vi "nipkg-updateControlFileMetadata.vi"() -> ()   [LabVIEW 2014, in "nipkg-build-system.lvlib"]
uses:
  nipkg-build-system.lvlib
  types/Package data.ctl
  <vilib>/Utility/file.llb/Read From Spreadsheet File (string).vi
  <vilib>/Utility/file.llb/Write To Spreadsheet File (string).vi
  <vilib>/Wiresmith Technology/LabVIEW CLI/CLI Class/CLI.lvclass
panel:
  out "error out":errorcluster
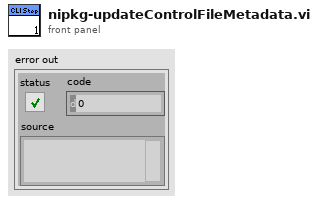
[diagram p1: front panel]
types:
  T1 = typedef "nipkg-build-system.lvlib/Package data.ctl" = cluster{"Package control file path":path, "Package metadata":string[]}
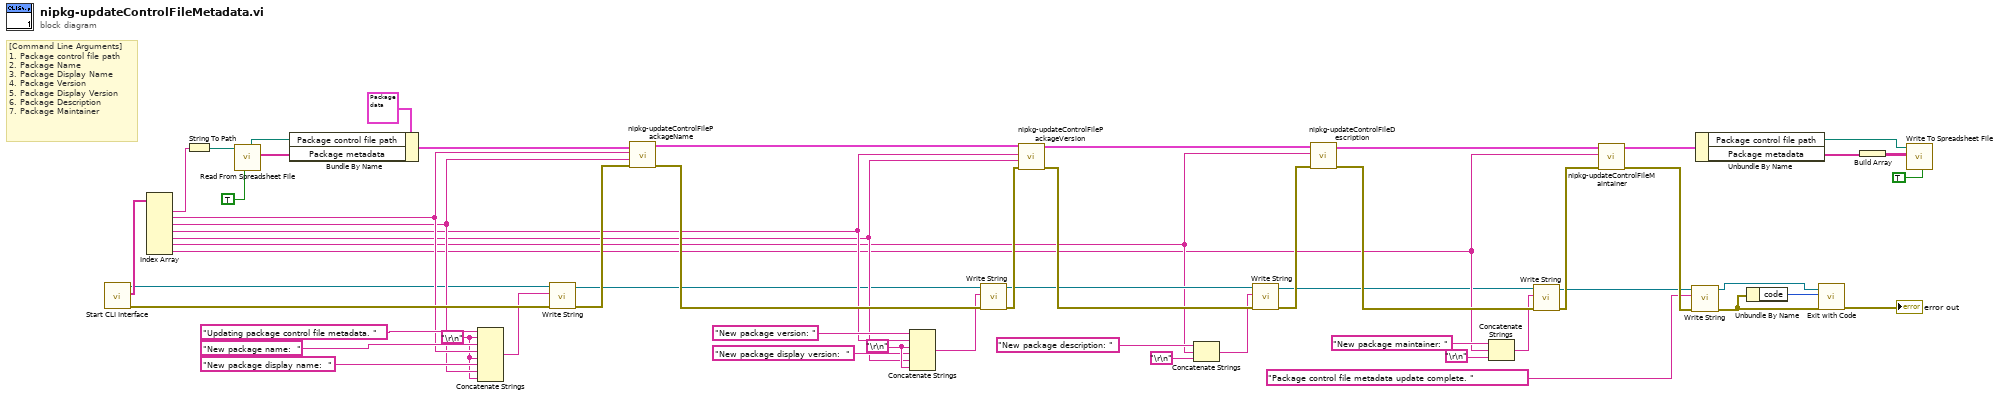
[diagram p0: block diagram]
diagram:
  w30 = "\r\n"
  w28 = "\r\n"
  # "[Command Line Arguments]\n1. Package control file path\n2. Package Name\n3. Package Display Name\n4. Package Version\n5. Package Display Version\n6. Package Description\n7. Package Maintainer"
  n1 = call <vilib>:"Start CLI Interface.vi"() -> ("error out"=w40:errorcluster, "Custom Parameters"=w43:string[], "CLI out"=w32:refnum<class "CLI.lvclass">)  [unwired: 9 in]
  n2 = Index Array(array=w43) -> (element #1=w42:string, element #2=w36:string, element #3=w34:string, element #4=w26:string, element #5=w25:string, element #6=w17:string, element #7=w12:string)  [unwired: 7 in]
  n3 = String To Path(string=w42) -> (path=w41:path)
  n4 = call-poly <vilib>:"Read From Spreadsheet File.vi"("transpose (no:F)"=TRUE, "file path (dialog if empty)"=w41) -> ("first row"=w54:string[], "new file path (Not A Path if cancelled)"=w48:path)  [unwired: 5 in, 3 out]
  n5 = Bundle By Name(cluster=T1 {"Package control file path"=path "C:/J/workspace/Waveform-Processing-CD/Package/Source/waveform-processing-custom-device/control/control", "Package metadata"=["Package: waveform-processing-custom-device"]} ("Package data"), "Package control file path"=w48, "Package metadata"=w54) -> (w53:T1)
  n6 = Concatenate Strings("Updating package control file metadata. ", w28, "New package name:  ", w36, w28, "New package display name:  ", w34, w28) -> (w33:string)
  n7 = call <vilib>:"Write String.vi"("error in (no error)"=w40, "Text to Write"=w33, "CLI in"=w32) -> ("error out"=w39:errorcluster, "CLI out"=w23:refnum<class "CLI.lvclass">)  [unwired: 7 in]
  n8 = call "nipkg-updateControlFilePackageName.vi"("error in (no error)"=w39, "New Package Display Name"=w34, "New Package Name"=w36, "Package data"=w53) -> ("error out"=w31:errorcluster, "Package data out"=w52:T1)  [unwired: 6 in]
  n9 = Concatenate Strings("New package version: ", w26, w30, "New package display version:  ", w25, w30) -> (w24:string)
  n10 = call <vilib>:"Write String.vi"("error in (no error)"=w31, "Text to Write"=w24, "CLI in"=w23) -> ("error out"=w22:errorcluster, "CLI out"=w20:refnum<class "CLI.lvclass">)  [unwired: 7 in]
  n11 = call "nipkg-updateControlFilePackageVersion.vi"("error in (no error)"=w22, "New Package Display Version"=w25, "New Package Version"=w26, "Package data"=w52) -> ("error out"=w21:errorcluster, "Package data out"=w51:T1)  [unwired: 6 in]
  n12 = Concatenate Strings("New package description: ", w17, "\r\n") -> (w9:string)
  n13 = call <vilib>:"Write String.vi"("error in (no error)"=w21, "Text to Write"=w9, "CLI in"=w20) -> ("error out"=w16:errorcluster, "CLI out"=w10:refnum<class "CLI.lvclass">)  [unwired: 7 in]
  n14 = call "nipkg-updateControlFileDescription.vi"("error in (no error)"=w16, "New Package Description"=w17, "Package data"=w51) -> ("error out"=w15:errorcluster, "Package data out"=w50:T1)  [unwired: 7 in]
  n15 = Concatenate Strings("New package maintainer: ", w12, "\r\n") -> (w8:string)
  n16 = call <vilib>:"Write String.vi"("error in (no error)"=w15, "Text to Write"=w8, "CLI in"=w10) -> ("error out"=w11:errorcluster, "CLI out"=w2:refnum<class "CLI.lvclass">)  [unwired: 7 in]
  n17 = call "nipkg-updateControlFileMaintainer.vi"("error in (no error)"=w11, "New Package Maintainer"=w12, "Package data"=w50) -> ("error out"=w6:errorcluster, "Package data out"=w49:T1)  [unwired: 7 in]
  n18 = call <vilib>:"Write String.vi"("error in (no error)"=w6, "Text to Write"="Package control file metadata update complete. ", "CLI in"=w2) -> ("error out"=w4:errorcluster, "CLI out"=w1:refnum<class "CLI.lvclass">)  [unwired: 7 in]
  n19 = Unbundle By Name(w49) -> ("Package control file path"=w44:path, "Package metadata"=w46:string[])
  n20 = Unbundle By Name(w4) -> ("code"=w3:i32)
  n21 = call <vilib>:"Exit with Code.vi"("error in (no error)"=w4, "Exit Code (0)"=w3, "CLI in"=w1) -> ("error out"=→"error out":errorcluster)  [unwired: 8 in]
  n22 = Build Array(w46) -> (w45:string[][])
  n23 = call-poly <vilib>:"Write To Spreadsheet File.vi"("transpose? (no:F)"=TRUE, "2D data"=w45, "file path (dialog if empty)"=w44) -> ()  [unwired: 5 in, 1 out]
